vi "Destroy.vi"(8 "error in (no error)":errorcluster, 11 "Animated Texture in":refnum<class "Animated Texture.lvclass">) -> (0 "error out":errorcluster)   [LabVIEW 2015, in "Animated Texture.lvclass"]
uses:
  Animated Texture.lvclass
  Animated Texture.lvclass/Animated Texture.ctl
  Texture/Texture.lvclass/Texture.ctl
  LabSDL2/Source/Libraries/LibSDL2 Wrapper/Destroy Texture.vi
  Texture/Texture.lvclass
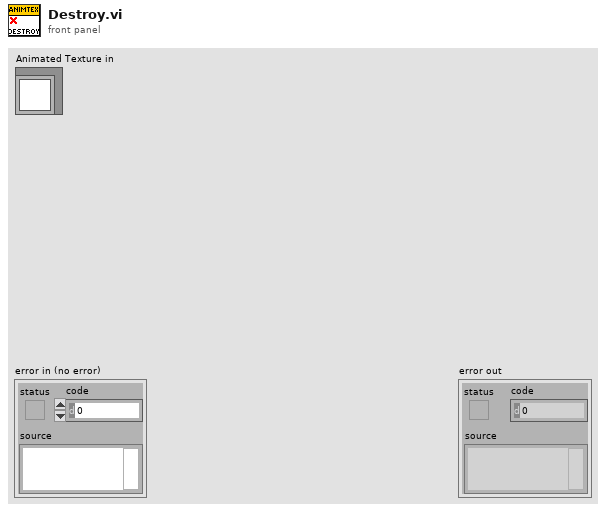
[diagram p1: front panel]
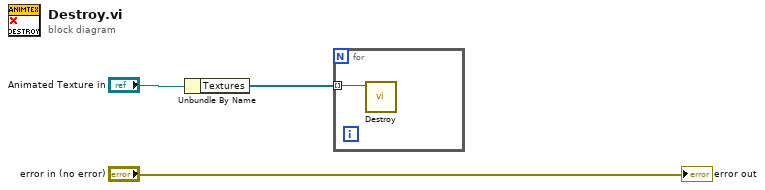
[diagram p0: block diagram]
diagram:
  n1 = Unbundle By Name("Animated Texture in") -> ("Textures"=w1:refnum<class "Texture.lvclass">[])
  n2 = for {
    tunnel: w1 -> [w4] mode=indexing
    n3 = call "Destroy.vi"("Texture in"=w4) -> ()  [unwired: 10 in, 1 out]
  }
  "error out" <- "error in (no error)"
